vi "Replace Outside Typedef Control.vi"(6 "dependent vis":path[](array[path]), 8 "error in":errorcluster, 9 "shared directory":path, 10 "non-library vi[]":string[](array[string]), 11 "measurement directory":path) -> (0 "error out":errorcluster)   [LabVIEW 2021, in "Multiple Converter.lvlib"]
uses:
  Multiple Converter.lvlib
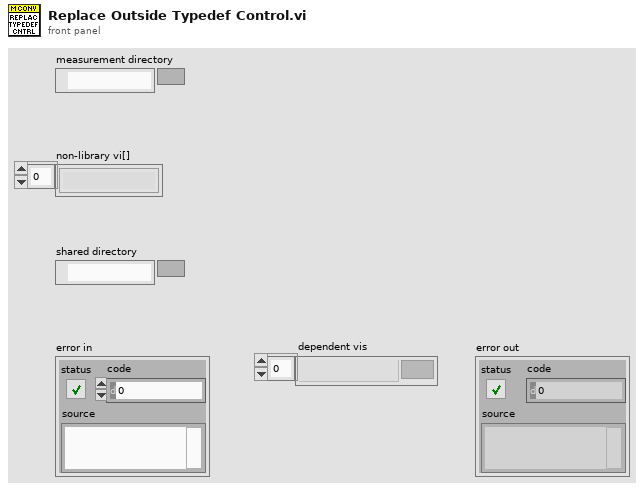
[diagram p1: front panel]
types:
  T1 = enum32{"not a typedef", "typedef", "strict typedef", "class private data"}
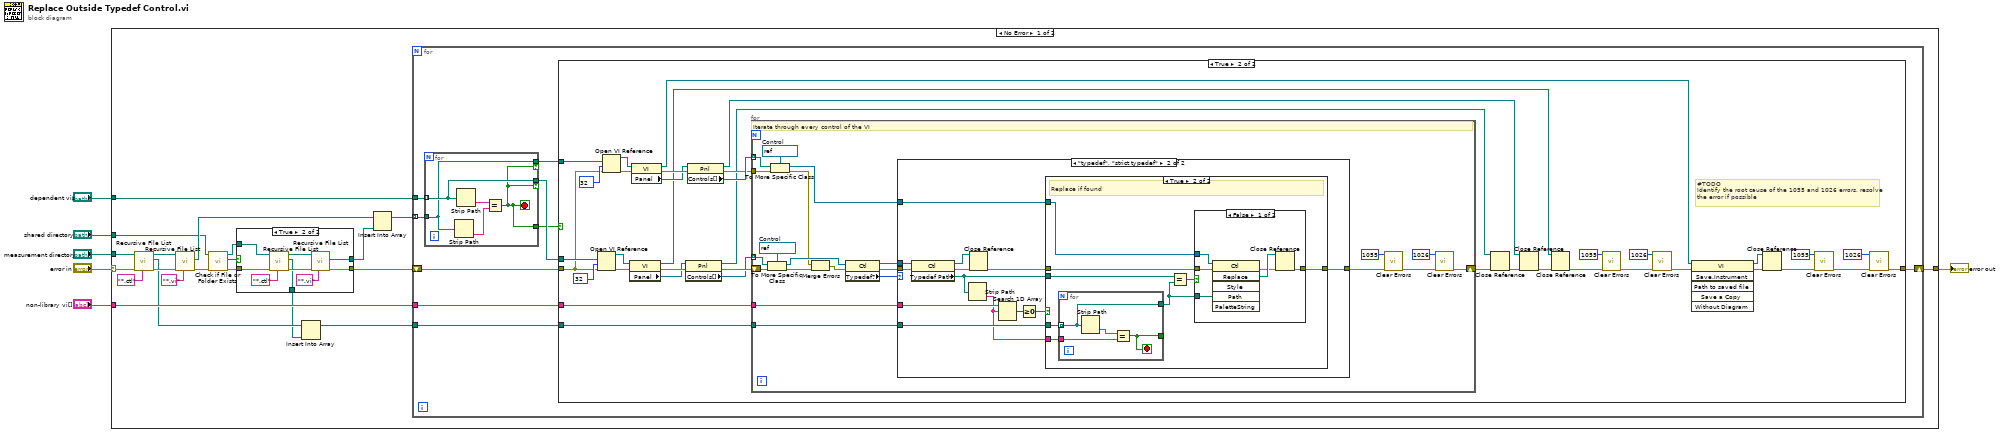
[diagram p0: block diagram]
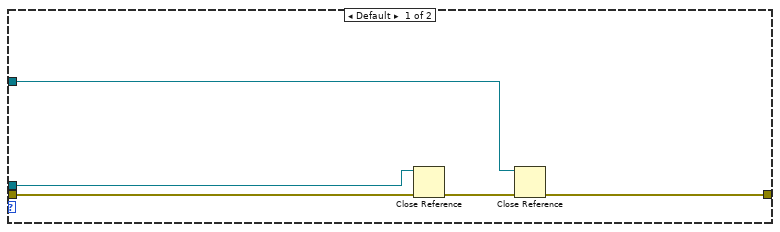
[diagram p3: hidden frame]
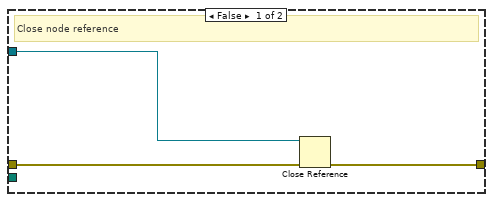
[diagram p4: hidden frame]
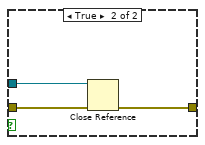
[diagram p5: hidden frame]
diagram:
  n1 = case shown="No Error" "error in" {
    selector: "error in" -> [w26 w154]
    tunnel: "non-library vi[]" -> [w27 _]
    tunnel: [w24 w154] -> w4
    tunnel: "measurement directory" -> [w22 _]
    tunnel: "shared directory" -> [w8 _]
    tunnel: "dependent vis" -> [w7 _]
    frame No Error {
      n2 = call <vilib>:"Recursive File List.vi"("pattern"="*.ctl", "error in (no error)"=w26, "Folder Path"=w22) -> ("error out"=w23:errorcluster, "All Files in Dir"=w19:path[], "dup Folder Path"=w21:path)  [unwired: 4 in, 2 out]
      n3 = call <vilib>:"Recursive File List.vi"("pattern"="*.vi", "error in (no error)"=w23, "Folder Path"=w21) -> ("error out"=w17:errorcluster, "All Files in Dir"=w16:path[])  [unwired: 4 in, 3 out]
      n4 = call <vilib>:"Check if File or Folder Exists.vi"("error in (no error)"=w17, "path"=w8) -> ("error out"=w11:errorcluster, "file or folder exists?"=w10:bool, "dup path"=w9:path)  [unwired: 7 in]
      n5 = case shown="True" w10 {
        tunnel: [w144 w149] -> w18
        tunnel: w11 -> [w144 w148]
        tunnel: [_ w147] -> w13
        tunnel: [_ w146] -> w12
        tunnel: w9 -> [_ w145]
        frame False {
        }
        frame True {
          n6 = call <vilib>:"Recursive File List.vi"("pattern"="*.ctl", "error in (no error)"=w148, "Folder Path"=w145) -> ("error out"=w151:errorcluster, "All Files in Dir"=w147:path[], "dup Folder Path"=w152:path)  [unwired: 4 in, 2 out]
          n7 = call <vilib>:"Recursive File List.vi"("pattern"="*.vi", "error in (no error)"=w151, "Folder Path"=w152) -> ("error out"=w149:errorcluster, "All Files in Dir"=w146:path[])  [unwired: 4 in, 3 out]
        }
      }
      n8 = Insert Into Array(array=w19, new element=w13) -> (w14:path[])  [unwired: 1 in]
      n9 = Insert Into Array(array=w16, new element=w12) -> (w15:path[])  [unwired: 1 in]
      n10 = for {
        tunnel: w14 -> [w36]
        tunnel: w27 -> [w35]
        tunnel: w15 -> [w33] mode=indexing
        shift-right: [w29] -> w24
        shift-left: w18 -> [w31]
        tunnel: w7 -> [w34]
        n11 = for {
          tunnel: w34 -> [w141] mode=indexing
          tunnel: w33 -> [w140]
          tunnel: [w141] -> w32 if=w139
          tunnel: [w140] -> w30 if=w139
          tunnel: [w139] -> w28
          stop <- w139 stop-if-true
          n12 = Strip Path(path=w140) -> (name=w142:string)  [unwired: 1 out]
          n13 = Strip Path(path=w141) -> (name=w143:string)  [unwired: 1 out]
          n14 = Equal?(x=w143, y=w142) -> (x = y?=w139:bool)
        }
        n15 = case shown="True" w28 {
          tunnel: w36 -> [_ w75]
          tunnel: w35 -> [_ w74]
          tunnel: w32 -> [_ w69]
          tunnel: w31 -> [w37 w67]
          tunnel: w30 -> [_ w66]
          tunnel: [w37 w49] -> w29
          frame False {
          }
          frame True {
            # "#TODO\nIdentify the root cause of the 1055 and 1026 errors, resolve \nthe error if possible"
            n16 = Open VI Reference(vi path=w69, options=32, error in (no error)=w67) -> (vi reference=w57:refnum<vi>, error out=w58:errorcluster)  [unwired: 3 in]
            n17 = Open VI Reference(vi path=w66, options=32, error in (no error)=w67) -> (vi reference=w64:refnum<vi>, error out=w59:errorcluster)  [unwired: 3 in]
            n18 = property class="VI"(reference=w57, error in=w58) -> (reference out=w39:refnum<vi>, error out=w60:errorcluster, "Panel"=w55:refnum<vi>)
            n19 = property class="VI"(reference=w64, error in=w59) -> (reference out=w38:refnum<vi>, error out=w63:errorcluster, "Panel"=w56:refnum<vi>)
            n20 = property class="Pnl"(reference=w55, error in=w60) -> (reference out=w41:refnum<vi>, error out=w54:errorcluster, "Controls[]"=w43:refnum<vi>[])
            n21 = property class="Pnl"(reference=w56, error in=w63) -> (reference out=w40:refnum<vi>, error out=w61:errorcluster, "Controls[]"=w62:refnum<vi>[])
            n22 = for {
              tunnel: w43 -> [w96] mode=indexing
              tunnel: w74 -> [w93]
              tunnel: w75 -> [w95]
              tunnel: w61 -> [w90]
              tunnel: w62 -> [w89] mode=indexing
              shift-right: [w76] -> w42
              shift-left: w54 -> [w81]
              w91 = refnum<vi> refnum  # Control
              w94 = refnum<vi> refnum  # Control
              # "Iterate through every control of the VI"
              n23 = To More Specific Class(target class=w94, reference=w96, error in=w81) -> (specific class reference=w92:refnum<vi>, error out=w86:errorcluster)
              n24 = To More Specific Class(target class=w91, reference=w89, error in=w90) -> (specific class reference=w88:refnum<vi>, error out=w85:errorcluster)
              n25 = Merge Errors(w85, w86) -> (w87:errorcluster)
              n26 = property class="Ctl"(reference=w92, error in=w87) -> (reference out=w83:refnum<vi>, error out=w84:errorcluster, "Typedef?"=w82:T1)
              n27 = case shown="\"typedef\", \"strict typedef\"" w82 {
                tunnel: w84 -> [w101 w103]
                tunnel: w83 -> [w99 w109]
                tunnel: [w98 w113] -> w80
                tunnel: w95 -> [_ w111]
                tunnel: w93 -> [_ w110]
                tunnel: w88 -> [w97 w104]
                frame Default {
                  n28 = Close Reference(reference=w99, error in (no error)=w101) -> (error out=w100:errorcluster)
                  n29 = Close Reference(reference=w97, error in (no error)=w100) -> (error out=w98:errorcluster)
                }
                frame "typedef", "strict typedef" {
                  n30 = property class="Ctl"(reference=w109, error in=w103) -> (reference out=w105:refnum<vi>, error out=w106:errorcluster, "Typedef Path"=w107:path)
                  n31 = Strip Path(path=w107) -> (name=w108:string)  [unwired: 1 out]
                  n32 = Close Reference(reference=w105, error in (no error)=w106) -> (error out=w102:errorcluster)
                  n33 = Search 1D Array(1D array=w110, element=w108) -> (index of element=w114:i32)  [unwired: 1 in]
                  n34 = Greater Or Equal To 0?(x=w114) -> (x >= 0?=w112:bool)
                  n35 = case shown="True" w112 {
                    tunnel: [w117 w123] -> w113
                    tunnel: w111 -> [_ w125]
                    tunnel: w108 -> [_ w124]
                    tunnel: w107 -> [_ w122]
                    tunnel: w104 -> [w116 w119]
                    tunnel: w102 -> [w115 w118]
                    frame False {
                      # "Close node reference"
                      n36 = Close Reference(reference=w116, error in (no error)=w115) -> (error out=w117:errorcluster)
                    }
                    frame True {
                      # "Replace if found"
                      n37 = for {
                        tunnel: w125 -> [w136] mode=indexing
                        tunnel: w124 -> [w137]
                        tunnel: [w136] -> w121
                        tunnel: [w135] -> _
                        stop <- w135 stop-if-true
                        n38 = Strip Path(path=w136) -> (name=w138:string)  [unwired: 1 out]
                        n39 = Equal?(x=w138, y=w137) -> (x = y?=w135:bool)
                      }
                      n40 = Equal?(x=w122, y=w121) -> (x = y?=w120:bool)
                      n41 = case shown="False" w120 {
                        tunnel: w118 -> [w131 w134]
                        tunnel: [w129 w133] -> w123
                        tunnel: w121 -> [w128 _]
                        tunnel: w119 -> [w126 w132]
                        frame False {
                          n42 = invoke class="Ctl" method="Replace"(reference=w126, error in=w131, "Path"=w128) -> (error out=w127:errorcluster, "Replace"=w130:refnum<vi>)  [unwired: 3 in, 4 out]
                          n43 = Close Reference(reference=w130, error in (no error)=w127) -> (error out=w129:errorcluster)
                        }
                        frame True {
                          n44 = Close Reference(reference=w132, error in (no error)=w134) -> (error out=w133:errorcluster)
                        }
                      }
                    }
                  }
                }
              }
              n45 = call <vilib>:"Clear Errors.vi"("error in (no error)"=w80, "specific error code to clear (0: all)"=1055) -> ("error out"=w79:errorcluster)  [unwired: 4 in, 1 out]
              n46 = call <vilib>:"Clear Errors.vi"("error in (no error)"=w79, "specific error code to clear (0: all)"=1026) -> ("error out"=w76:errorcluster)  [unwired: 4 in, 1 out]
            }
            n47 = Close Reference(reference=w41, error in (no error)=w42) -> (error out=w53:errorcluster)
            n48 = Close Reference(reference=w40, error in (no error)=w53) -> (error out=w52:errorcluster)
            n49 = Close Reference(reference=w39, error in (no error)=w52) -> (error out=w65:errorcluster)
            n50 = call <vilib>:"Clear Errors.vi"("error in (no error)"=w65, "specific error code to clear (0: all)"=1055) -> ("error out"=w47:errorcluster)  [unwired: 4 in, 1 out]
            n51 = call <vilib>:"Clear Errors.vi"("error in (no error)"=w47, "specific error code to clear (0: all)"=1026) -> ("error out"=w51:errorcluster)  [unwired: 4 in, 1 out]
            n52 = invoke class="VI" method="Save.Instrument"(reference=w38, error in=w51) -> (reference out=w71:refnum<vi>, error out=w72:errorcluster)  [unwired: 4 in, 4 out]
            n53 = Close Reference(reference=w71, error in (no error)=w72) -> (error out=w73:errorcluster)
            n54 = call <vilib>:"Clear Errors.vi"("error in (no error)"=w73, "specific error code to clear (0: all)"=1055) -> ("error out"=w45:errorcluster)  [unwired: 4 in, 1 out]
            n55 = call <vilib>:"Clear Errors.vi"("error in (no error)"=w45, "specific error code to clear (0: all)"=1026) -> ("error out"=w49:errorcluster)  [unwired: 4 in, 1 out]
          }
        }
      }
    }
    frame Error {
    }
  }
  "error out" <- w4
